vi "AlarmGetRulesResponse_Parse.vi"(8 "error in (no error)":errorcluster, 11 "Message":T9) -> (0 "error out":errorcluster, 1 "Body":T1, 2 "Header":T8, 3 "AlarmGetRulesResponse":T7)   [LabVIEW 2017]
uses:
  <vilib>/addons/InsightCM/MessageBus/Base/controls/Message.ctl
  <vilib>/addons/InsightCM/MessageBus/Base/controls/MessageHeader.ctl
  <vilib>/addons/InsightCM/MessageBus/Base/controls/KeyValuePair.ctl
  <vilib>/addons/InsightCM/MessageBus/MessageLibrary/Alarm/controls/AlarmGetRulesResponse.ctl
  <vilib>/addons/InsightCM/MessageBus/MessageLibrary/Alarm/controls/AlarmGetRulesResponseBody.ctl
  <vilib>/addons/InsightCM/MessageBus/Base/controls/AlarmRule.ctl
  <vilib>/addons/InsightCM/MessageBus/Base/controls/AlarmTrigger.ctl
  <vilib>/addons/InsightCM/MessageBus/Base/controls/AlarmCondition.ctl
  <vilib>/addons/InsightCM/MessageBus/Base/controls/AlarmAction.ctl
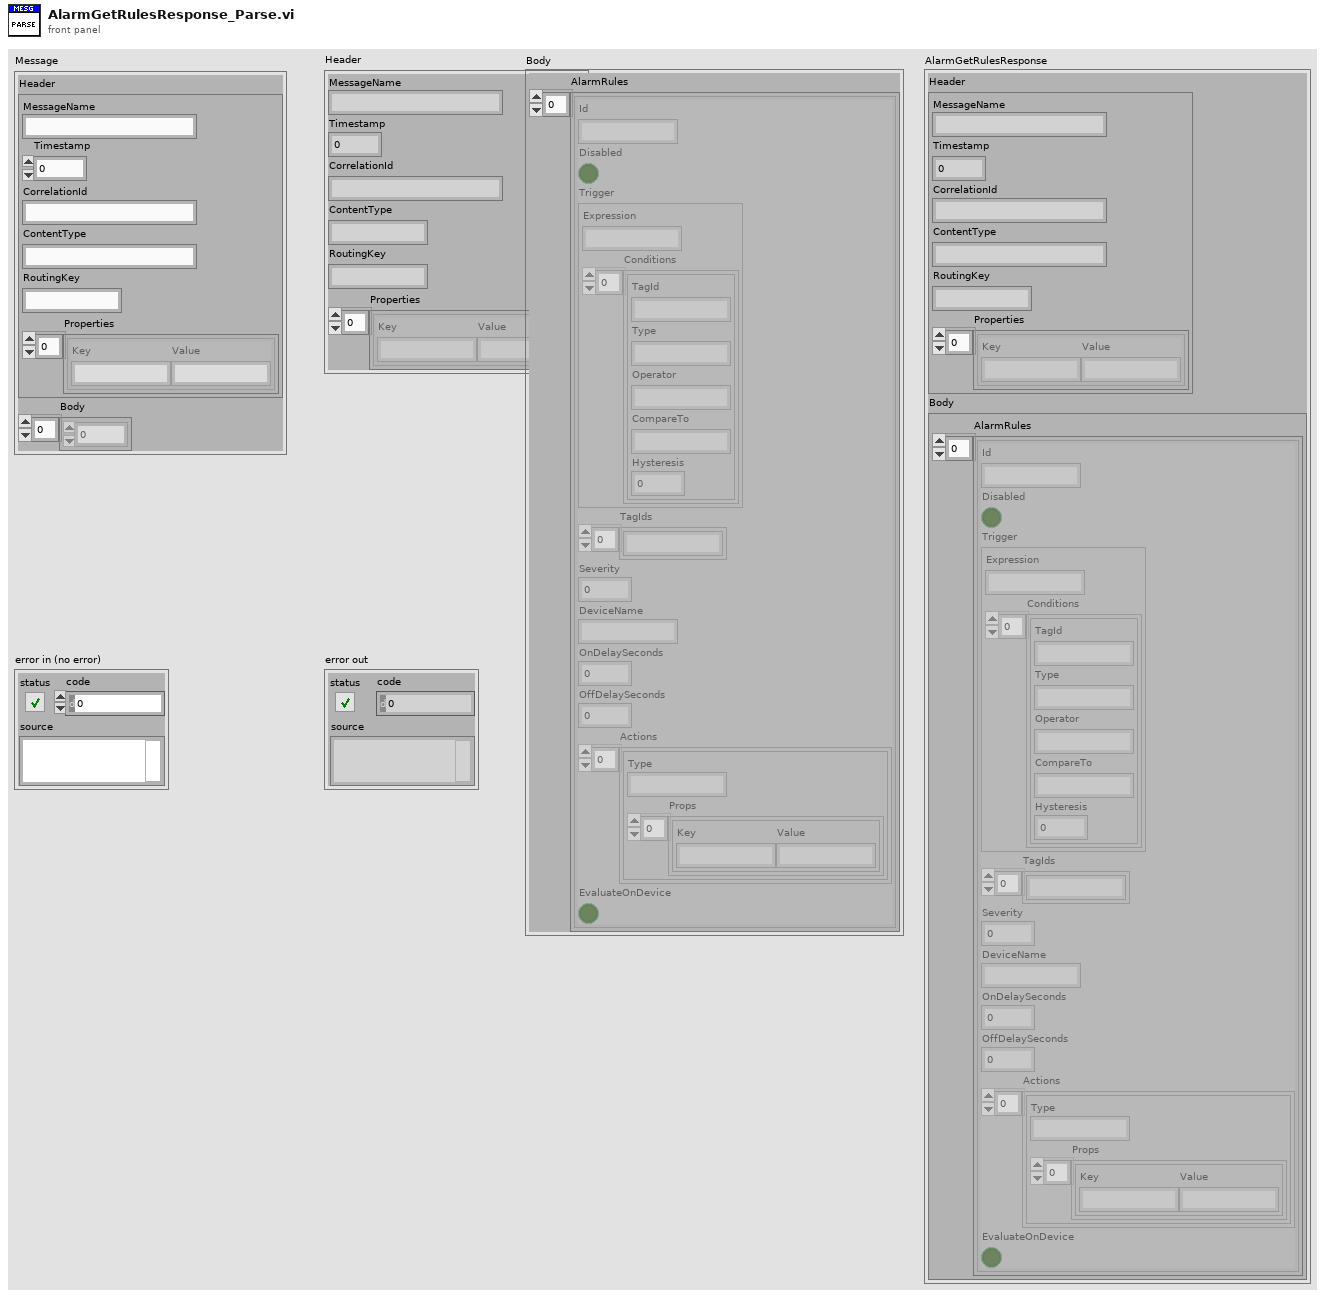
[diagram p1: front panel]
types:
  T1 = typedef "AlarmGetRulesResponseBody.ctl" = cluster{"AlarmRules":T2[]}
  T2 = typedef "AlarmRule.ctl" = cluster{"Id":string, "Disabled":bool, "Trigger":T3, "TagIds":string[], "Severity":i32, "DeviceName":string, "OnDelaySeconds":dbl, "OffDelaySeconds":dbl, "Actions":T5[], "EvaluateOnDevice":bool}
  T3 = typedef "AlarmTrigger.ctl" = cluster{"Expression":string, "Conditions":T4[]}
  T4 = typedef "AlarmCondition.ctl" = cluster{"TagId":string, "Type":string, "Operator":string, "CompareTo":string, "Hysteresis":dbl}
  T5 = typedef "AlarmAction.ctl" = cluster{"Type":string, "Props":T6[]}
  T6 = typedef "KeyValuePair.ctl" = cluster{"Key":string, "Value":string}
  T7 = typedef "AlarmGetRulesResponse.ctl" = cluster{"Header":T8, "Body":T1}
  T8 = typedef "MessageHeader.ctl" = cluster{"MessageName":string, "Timestamp":i64, "CorrelationId":string, "ContentType":string, "RoutingKey":string, "Properties":T6[]}
  T9 = typedef "Message.ctl" = cluster{"Header":T8, "Body":u8[]}
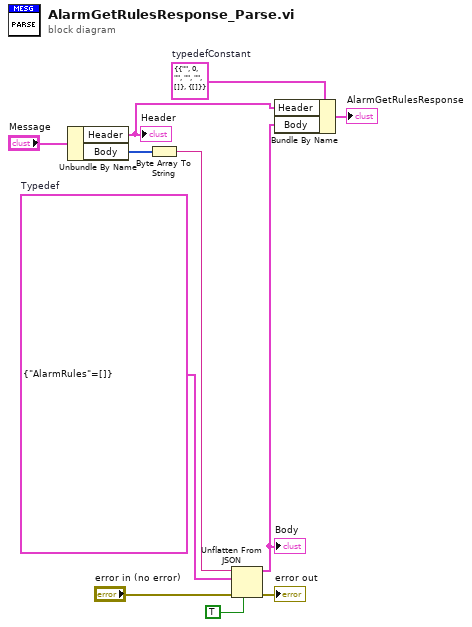
[diagram p0: block diagram]
diagram:
  w3 = T7 {"Header"={"MessageName"="", "Timestamp"=0, "CorrelationId"="", "ContentType"="", "RoutingKey"="", "Properties"=[]}, "Body"={"AlarmRules"=[]}}  # typedefConstant
  w7 = T1 {"AlarmRules"=[]}  # Typedef
  n1 = Unbundle By Name("Message") -> ("Header"=w9:T8, "Body"=w1:u8[])
  "Header" <- w9
  n2 = Byte Array To String(unsigned byte array=w1) -> (string=w6:string)
  n3 = Unflatten From JSON(JSON string=w6, type and defaults=w7, default null elements? (F)=TRUE, error in (no error)="error in (no error)") -> (value=w5:T1, error out=→"error out":errorcluster)  [unwired: 3 in]
  "Body" <- w5
  n4 = Bundle By Name(cluster=w3, "Header"=w9, "Body"=w5) -> (→"AlarmGetRulesResponse":T7)
